vi "robotModelTest2.vi"(0 "Communication in":refnum<class "Communication.lvclass">, 1 "Game in":refnum<class "Game.lvclass">, 3 "V_sent":dbl, 4 "V_sample":dbl, 5 "error in (no error)":errorcluster, 6 "id":i32, 7 "Samples":dbl, 8 "RobotModelFolder":string, 10 "Start":bool=TRUE, 11 "delta":dbl, 12 "replace active":bool, 13 "grSIM replacement.robots":T1[](array[typedef])) -> (14 "Game out":refnum<class "Game.lvclass">, 15 "TestTeam":refnum<class "Ally.lvclass">, 17 "Replace":bool, 18 "State":T2 {"progress" scale=0.0..100.0}, 19 "error out":errorcluster)   [LabVIEW 2021, in "Game.lvclass"]
uses:
  Game.lvclass
  Controls/RobotModel.ctl
  Communication_class/Communication.lvclass
  Ally_class/Ally.lvclass
  D:/RoboIme/horie/SSL_AI/Team_class/Team.lvclass
  Controls/RobotModelTestState.ctl
  Communication_class/Paths/grSim Packet Command UDP Test Folder/grSim/grSim RobotReplacement.ctl
  Game.lvclass/Game.ctl
  Team_class/Team.lvclass/Team.ctl
  Object_class/Object.lvclass/Object.ctl
  Robot_class/Robot.lvclass/Robot.ctl
  Object_class/Read x.vi
  Object_class/Read y.vi
  Read TestTeam.vi
  Read AllyRef.vi
  Team_class/Read RobotRef.vi
  Team_class/Write RobotRef.vi
  Robot_class/Read est_v_tang.vi
  Robot_class/Robot.lvclass
  D:/RoboIme/horie/SSL_AI/Object_class/Object.lvclass
  Utilities_class/Utilities.lvclass
panel:
  out "output array":dbl[](array[numeric])
  out "Mean":T3[](array[typedef])
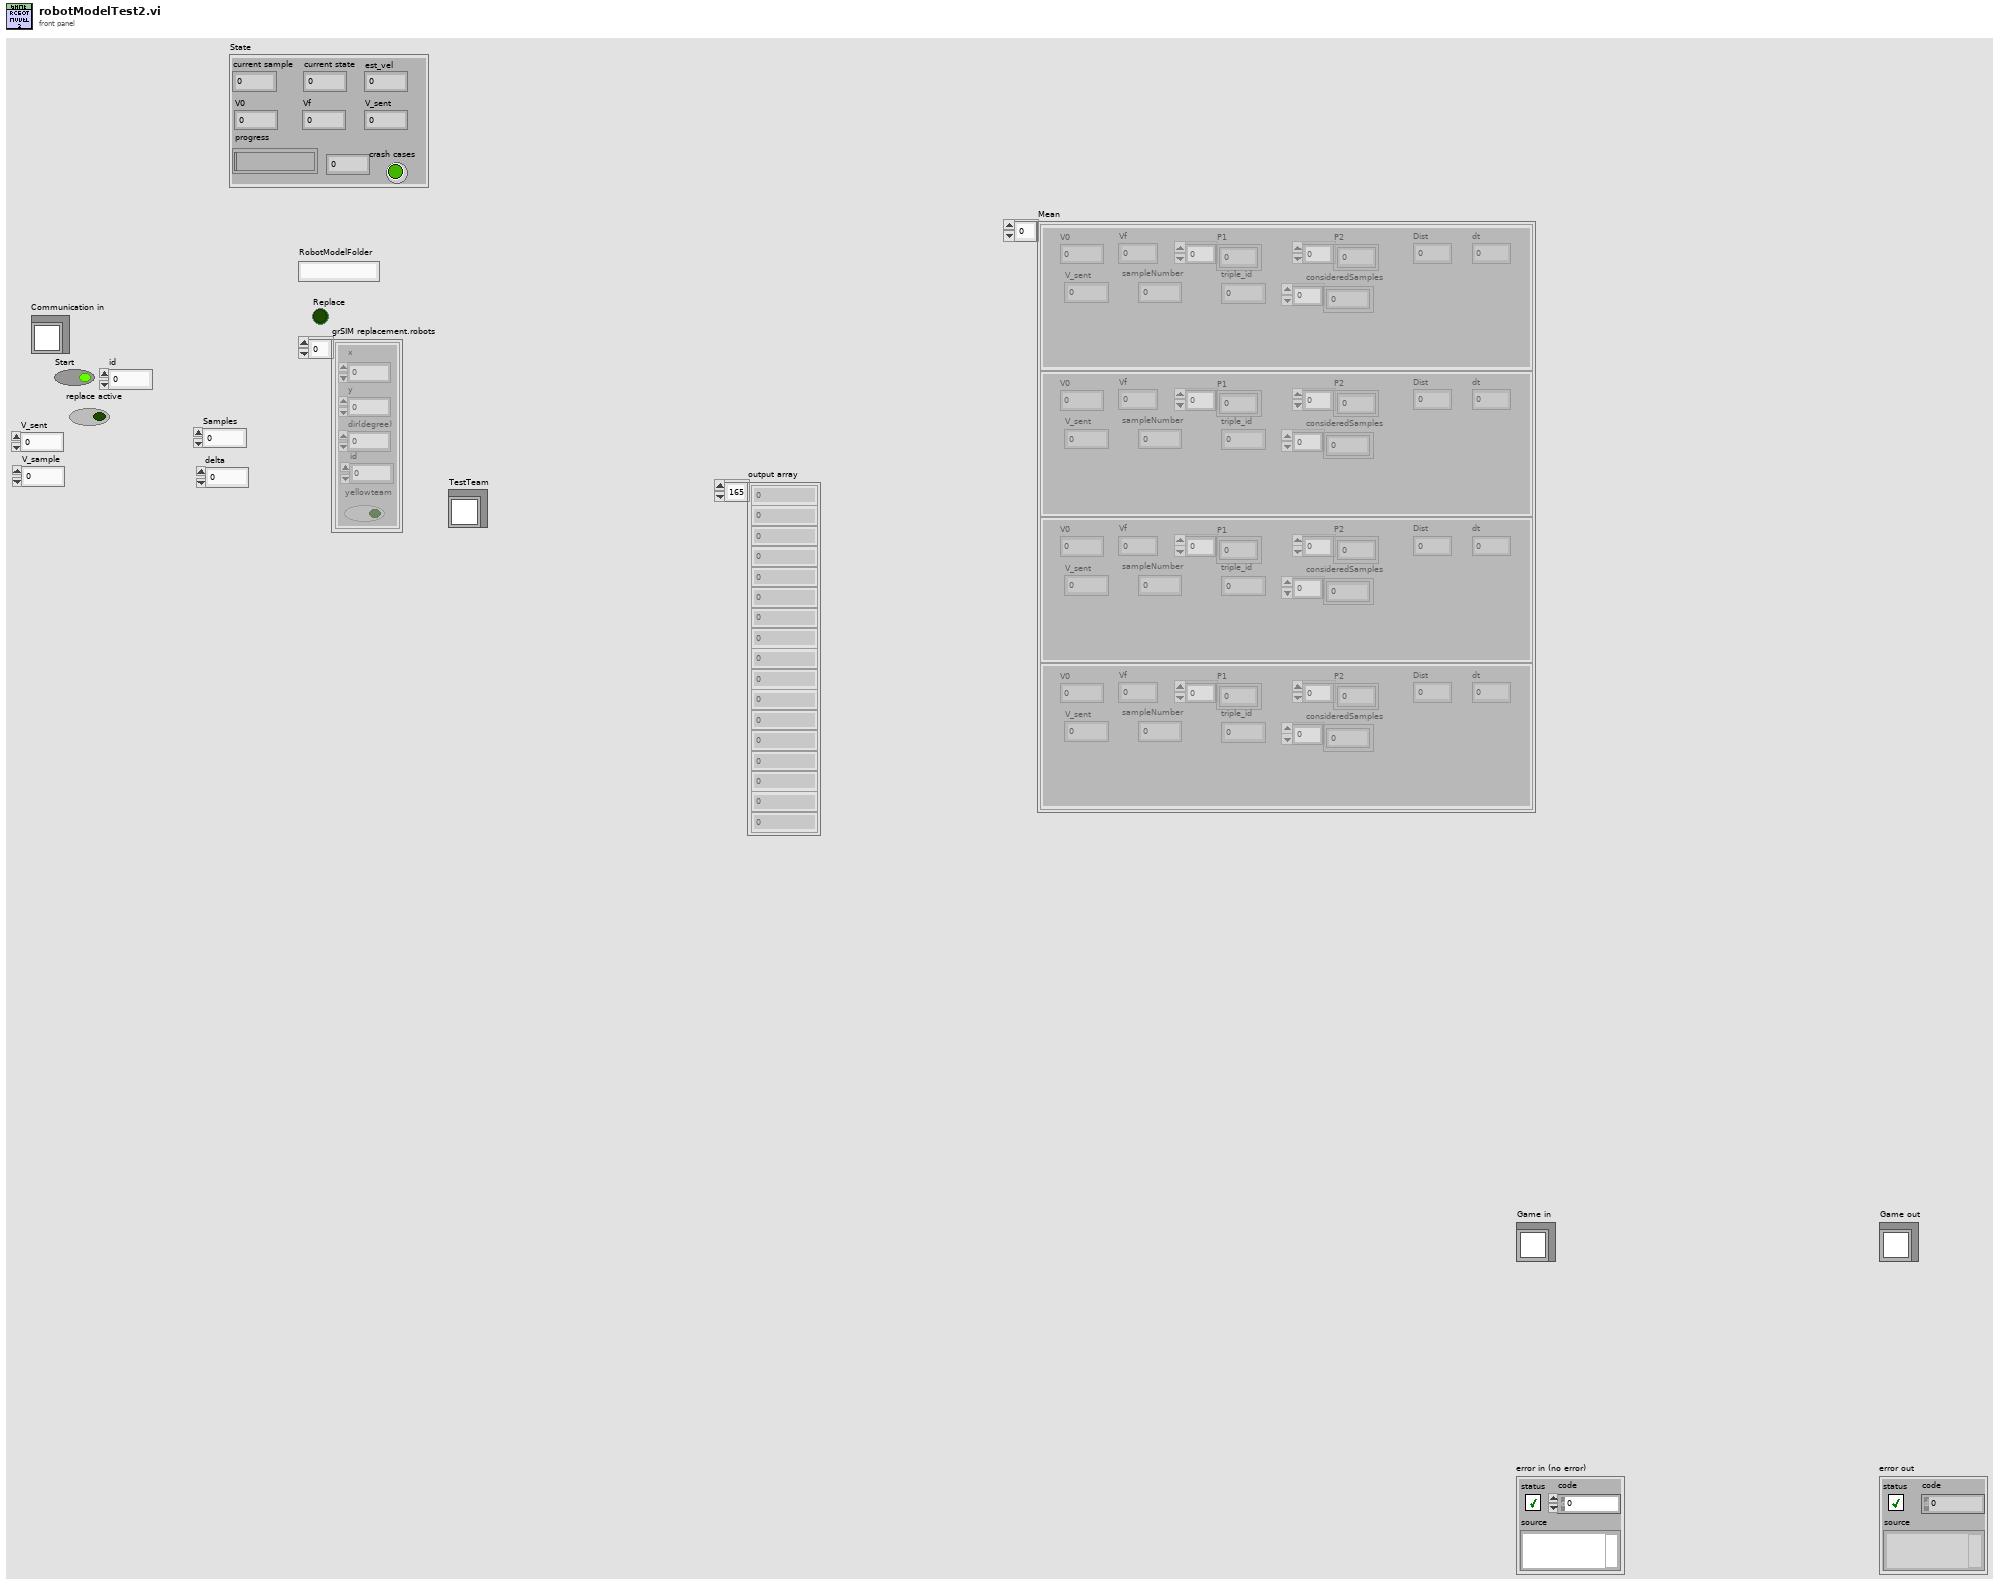
[diagram p1: front panel]
types:
  T1 = typedef "grSim RobotReplacement.ctl" = cluster{"x":dbl, "y":dbl, "dir(degree)":dbl, "yellowteam":bool, "id":u32}
  T2 = typedef "RobotModelTestState.ctl" = cluster{"current sample":i32, "V0":dbl, "Vf":dbl, "progress":dbl, "current state":i32, "est_vel":dbl, "V_sent":dbl, "crash cases":bool}
  T3 = typedef "RobotModel.ctl" = cluster{"V0":dbl, "Vf":dbl, "Dist":dbl, "dt":dbl, "P1":dbl[], "P2":dbl[], "V_sent":dbl, "sampleNumber":i32, "triple_id":i32, "consideredSamples":dbl[]}
  T4 = typedef "RobotModelAllInformation.ctl" = cluster{"distance":dbl, "lastRobotPosition":dbl[], "timestampOn2ndStateStart":timestamp, "sampleCount":i32, "stateInMachine":i32, "crashCases":T5[], "lastEstVel":dbl, "IdealVelocities":dbl[][], "RealVelocities":dbl[][], "testFinished?":bool, "RobotModelArray":T6}
  T5 = typedef "RobotModelTestCrashCase.ctl" = cluster{"real_V0":dbl, "real_Vf":dbl, "V_sent":dbl, "est_vel":dbl, "ideal_V0":dbl, "ideal_Vf":dbl}
  T6 = typedef "robotModelArray.ctl" = T3[]
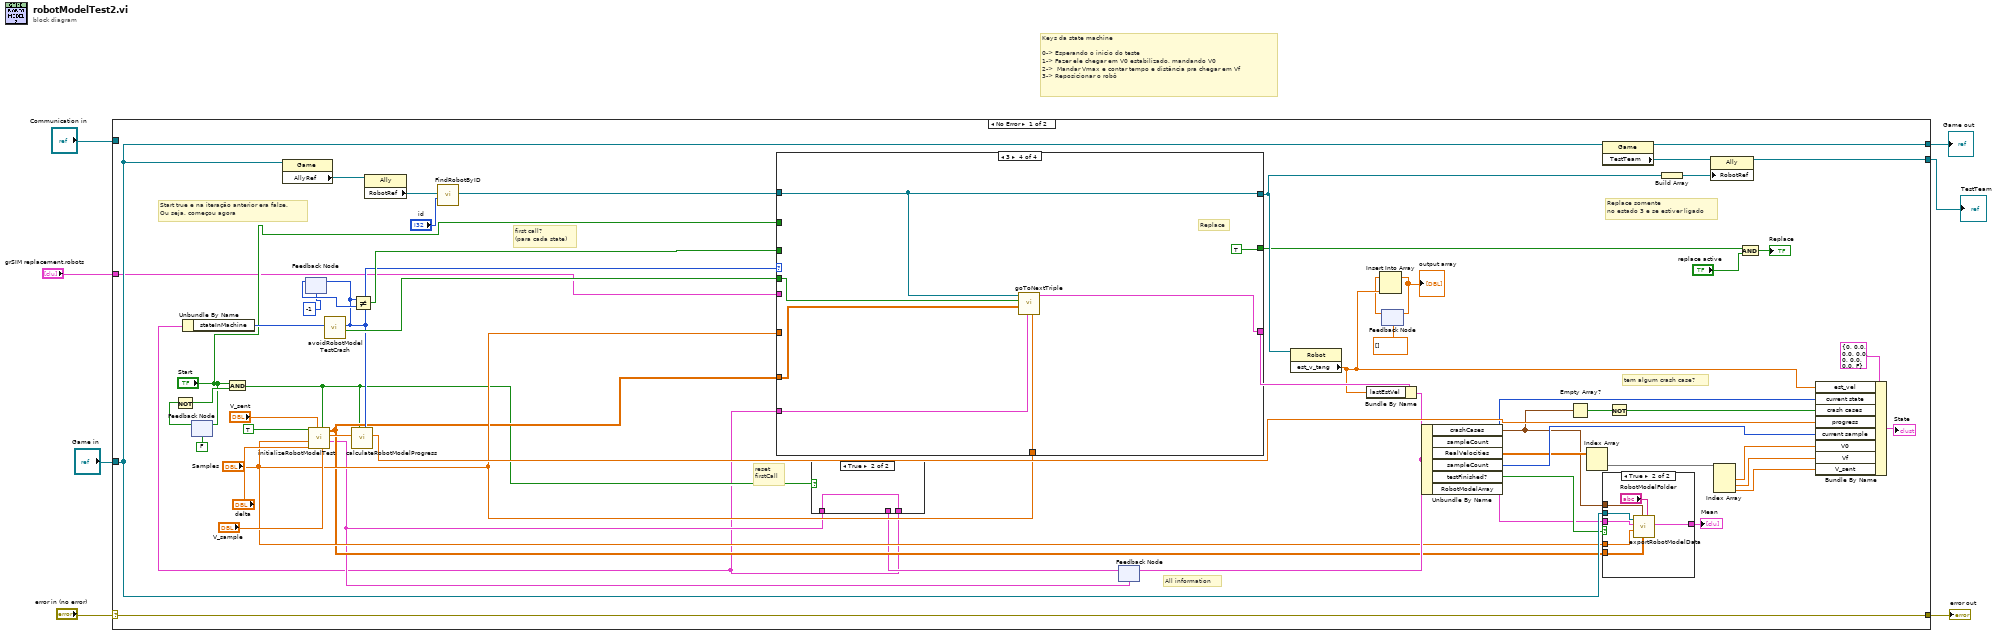
[diagram p0: block diagram]
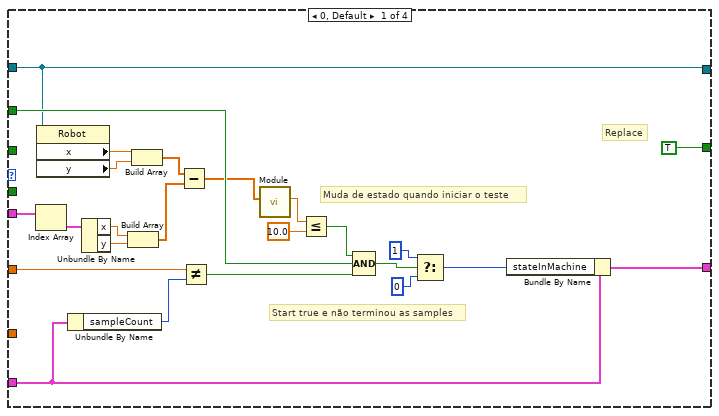
[diagram p3: hidden frame]
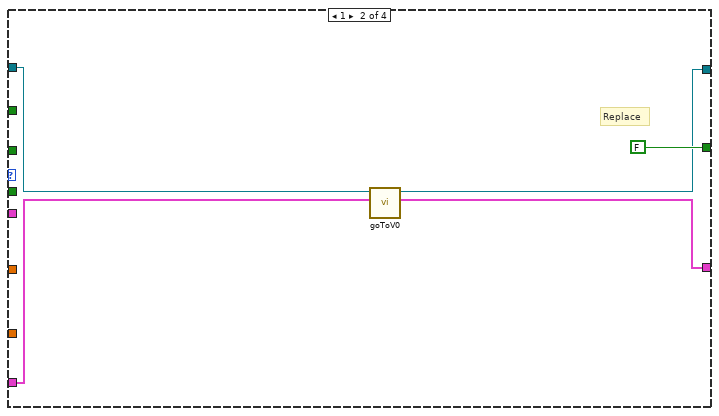
[diagram p4: hidden frame]
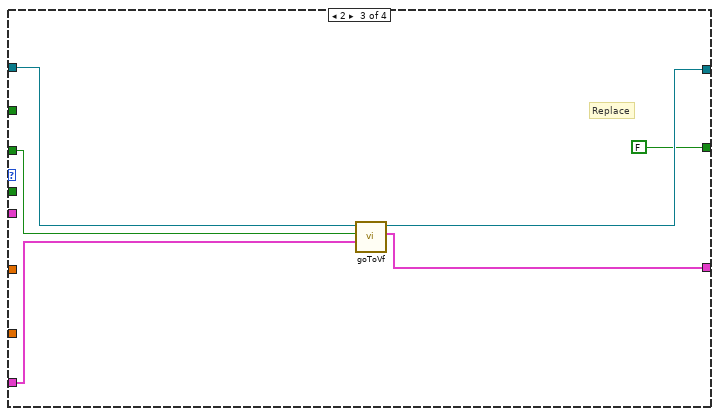
[diagram p5: hidden frame]
diagram:
  # "Keys da state machine\n\n0-> Esperando o inicio do teste\n1-> Fazer ele chegar em V0 estabilizado, mandando V0\n2->  Mandar Vmax e contar tempo e distância pra chegar em Vf \n3-> Reposicionar o robô"
  n1 = case shown="No Error" "error in (no error)" {
    selector: "error in (no error)" -> [w65 w117]
    tunnel: [w65 w117] -> w6
    tunnel: "Game in" -> [w48 _]
    tunnel: [w51 _] -> w4
    tunnel: [w52 _] -> w3
    tunnel: "Communication in" -> [_ _]
    tunnel: "grSIM replacement.robots" -> [w14 _]
    frame No Error {
      # "reset\nfirstCall"
      # "All information"
      # "Start true e na iteração anterior era false.\nOu seja, começou agora"
      # "tem algum crash case?"
      # "first call?\n(para cada state)"
      # "Replace somente\nno estado 3 e se estiver ligado"
      n2 = feedback #1(FALSE ("start")) -> (w39:bool)
      n3 = Not(x=w39) -> (.not. x?=w40:bool)
      n4 = feedback-in #1("Start") -> ()
      n5 = And(x="Start", y=w40) -> (x .and. y?=w12:bool)
      n6 = property class="Game"(reference=w48) -> ("AllyRef"=w62:refnum<class "Ally.lvclass">)  [unwired: 1 in, 2 out]
      n7 = feedback #2(-1) -> (w59:i32)
      n8 = call "initializeRobotModelTest.vi"("V_sample"="V_sample", "start"=w12, "delta"="delta", "V_sent"="V_sent", "Samples"="Samples", "fixed_V_sent?"=TRUE) -> ("RobotModelAllInformation out"=w11:T4, "totalNumberOfTests"=w32:dbl, "triples (V0, Vf, V_sent)"=w24:dbl[][])  [unwired: 3 in]
      n9 = property class="Ally"(reference=w62) -> ("RobotRef"=w61:refnum<class "Robot.lvclass">[])  [unwired: 1 in, 2 out]
      n10 = call "FindRobotByID.vi"("id"="id", "RobotRef"=w61) -> ("Robot"=w60:refnum<class "Robot.lvclass">)  [unwired: 6 in, 3 out]
      n11 = feedback #3(w11) -> (w10:T4)
      n12 = case shown="True" w12 {
        tunnel: [w66 w67] -> w9
        tunnel: w11 -> [_ w67]
        tunnel: w10 -> [w66 _]
        frame False {
        }
        frame True {
        }
      }
      n13 = Unbundle By Name(w9) -> ("stateInMachine"=w41:i32)
      n14 = call "avoidRobotModelTestCrash.vi"("state in"=w41) -> ("crash?"=w46:bool, "state out"=w36:i32)  [unwired: 7 in, 2 out]
      n15 = feedback-in #2(w36) -> ()
      n16 = call "calculateRobotModelProgress.vi"("current state"=w36, "start"=w12, "totalNumerOfTests"=w32) -> ("progress"=w47:dbl)  [unwired: 8 in]
      n17 = Not Equal?(x=w36, y=w59) -> (x != y?=w57:bool)
      n18 = case shown="3" w36 {
        tunnel: "Start" -> [w90 _ _ _]
        tunnel: w60 -> [w80 w95 w100 w107]
        tunnel: [w80 w94 w102 w107] -> w56
        tunnel: [TRUE FALSE FALSE TRUE] -> w23
        tunnel: w57 -> [_ _ w98 _]
        tunnel: "Samples" -> [w87 _ _ _]
        tunnel: w46 -> [_ _ _ w108]
        tunnel: w9 -> [w83 w92 w97 w106]
        tunnel: [w84 w93 w99 w105] -> w43
        tunnel: "Samples" -> [_ _ _ w103]
        tunnel: w24 -> [_ _ _ w104]
        tunnel: w14 -> [w76 _ _ _]
        frame 0, Default {
          # "Start true e não terminou as samples"
          # "Replace"
          # "Muda de estado quando iniciar o teste"
          n19 = Index Array(array=w76) -> (element=w75:T1)  [unwired: 1 in]
          n20 = property class="Robot"(reference=w80) -> ("x"=w79:dbl, "y"=w78:dbl)  [unwired: 1 in, 2 out]
          n21 = Unbundle By Name(w83) -> ("sampleCount"=w82:i32)
          n22 = Unbundle By Name(w75) -> ("x"=w74:dbl, "y"=w73:dbl)
          n23 = Build Array(w74, w73) -> (w72:dbl[])
          n24 = Build Array(w79, w78) -> (w77:dbl[])
          n25 = Subtract(x=w77, y=w72) -> (x-y=w71:dbl[])
          n26 = Not Equal?(x=w87, y=w82) -> (x != y?=w86:bool)
          n27 = call "Module.vi"("2D vector"=w71) -> ("Modulo"=w70:dbl)  [unwired: 8 in, 2 out]
          n28 = Less Or Equal?(x=w70, y=10.0) -> (x <= y?=w68:bool)
          n29 = Compound Arithmetic op=AND(w68, w90, w86) -> (w89:bool)
          n30 = Select(t=1, s=w89, f=0) -> (s? t:f=w85:i32)
          n31 = Bundle By Name(cluster=w83, "stateInMachine"=w85) -> (w84:T4)
        }
        frame 1 {
          # "Replace"
          n32 = call "goToV0.vi"("RobotModelAllInformation in"=w92, "Robot in"=w95) -> ("RobotModelAllInformation out"=w93:T4, "Robot out"=w94:refnum<class "Robot.lvclass">)  [unwired: 8 in]
        }
        frame 2 {
          # "Replace"
          n33 = call "goToVf.vi"("RobotModelAllInformation in"=w97, "firstCall?"=w98, "Robot in"=w100) -> ("RobotModelAllInformation out"=w99:T4, "Robot out"=w102:refnum<class "Robot.lvclass">)  [unwired: 7 in]
        }
        frame 3 {
          # "Replace"
          n34 = call "goToNextTriple.vi"("Samples"=w103, "RobotModelAllInformation in"=w106, "triples (V0, Vf, V_sent)"=w104, "crash?"=w108, "Robot in"=w107) -> ("RobotModelAllInformation out"=w105:T4)  [unwired: 6 in]
        }
      }
      n35 = property class="Robot"(reference=w56) -> ("est_v_tang"=w18:dbl)  [unwired: 1 in, 2 out]
      n36 = Bundle By Name(cluster=w43, "lastEstVel"=w18) -> (w42:T4)
      n37 = feedback-in #3(w42) -> ()
      n38 = feedback #4(dbl[] []) -> (w16:dbl[])
      n39 = Insert Into Array(array=w16, new element=w18) -> (w17:dbl[])  [unwired: 1 in]
      "output array" <- w17
      n40 = feedback-in #4(w17) -> ()
      n41 = Unbundle By Name(w42) -> ("crashCases"=w21:T5[], "sampleCount"=w19:i32, "RealVelocities"=w29:dbl[][], "sampleCount"=w44:i32, "testFinished?"=w13:bool, "RobotModelArray"=w8:T6)
      n42 = Empty Array?(array=w21) -> (empty?=w45:bool)
      n43 = Index Array(array=w29) -> (element=w28:dbl[])  [unwired: 2 in]
      n44 = case shown="True" w13 {
        tunnel: "Samples" -> [_ w114]
        tunnel: w8 -> [_ w116]
        tunnel: w48 -> [_ w115]
        tunnel: [_ w113] -> w53
        tunnel: w21 -> [_ w112]
        tunnel: w24 -> [_ w111]
        frame False {
        }
        frame True {
          n45 = call "exportRobotModelData.vi"("RobotModelFolder"="RobotModelFolder", "triples (V0, Vf, V_sent)"=w111, "CrashCases"=w112, "Samples"=w114, "RobotModelArray"=w116, "Game in"=w115) -> ("Mean"=w113:T3[])  [unwired: 2 in, 3 out]
        }
      }
      "Mean" <- w53
      n46 = property class="Game"(reference=w48) -> (reference out=w51:refnum<class "Game.lvclass">, "TestTeam"=w54:refnum<class "Ally.lvclass">)  [unwired: 1 in, 1 out]
      n47 = Not(x=w45) -> (.not. x?=w20:bool)
      n48 = Build Array(w56) -> (w55:refnum<class "Robot.lvclass">[])
      n49 = property class="Ally"(reference=w54, "RobotRef"=w55) -> (reference out=w52:refnum<class "Ally.lvclass">)  [unwired: 1 in, 1 out]
      n50 = Index Array(array=w28) -> (element #1=w27:dbl, element #2=w26:dbl, element #3=w25:dbl)  [unwired: 3 in]
      n51 = And(x=w23, y="replace active") -> (x .and. y?=→"Replace":bool)
      n52 = Bundle By Name(cluster=T2 {"current sample"=0, "V0"=0.0, "Vf"=0.0, "progress"=0.0, "current state"=0, "est_vel"=0.0, "V_sent"=0.0, "crash cases"=FALSE} ("State"), "est_vel"=w18, "current state"=w19, "crash cases"=w20, "progress"=w47, "current sample"=w44, "V0"=w27, "Vf"=w26, "V_sent"=w25) -> (→"State":T2)
    }
    frame Error {
    }
  }
  "error out" <- w6
  "Game out" <- w4
  "TestTeam" <- w3
